vi "Delete Data DVR.vi"(8 "error in (no error)":errorcluster, 11 "Data DVR in":refnum<data-value>) -> (0 "error out":errorcluster, 3 "Data out":refnum<class "Data.lvclass">)   [LabVIEW 2013, in "MDSplus.lvlib" / "Data.lvclass"]
uses:
  <vilib>/MDSplus/Classes/Data_Class/Data.lvclass
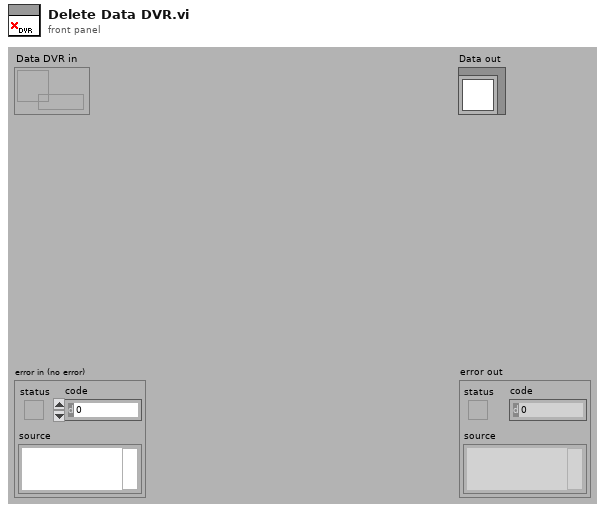
[diagram p1: front panel]
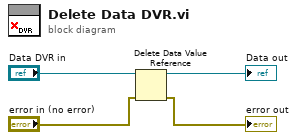
[diagram p0: block diagram]
diagram:
  n1 = Delete Data Value Reference(data value reference="Data DVR in", error in="error in (no error)") -> (data value=→"Data out":refnum<class "Data.lvclass">, error out=→"error out":errorcluster)
